vi "Configure Numeric Control.vi"(8 "error in":errorcluster, 10 "control":refnum<vi>, 11 "Value in":refnum<class "Value.lvclass">) -> (0 "error out":errorcluster, 3 "Value out":refnum<class "Value.lvclass">)   [LabVIEW 2020, in "Value.lvlib" / "Value.lvclass"]
doc: "Set the format, precision and limits of the control from the value metadata"
uses:
  Value.lvclass
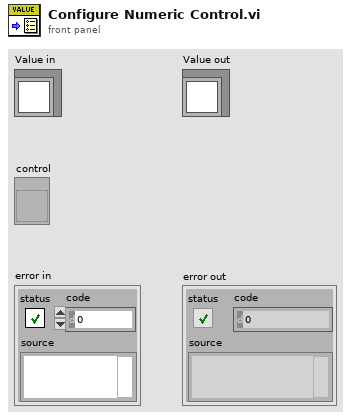
[diagram p1: front panel]
types:
  T1 = typedef "Value.lvlib/Display Metadata.ctl" = cluster{"Limit Low":dbl, "Limit High":dbl, "Description":string, "Units":string, "Precision":i32, "Form":enum32{"Default", "String", "Binary", "Decimal", "Hex", "Exponential", "Engineering"}}
  T2 = enum32{"Default", "String", "Binary", "Decimal", "Hex", "Exponential", "Engineering"}
  T3 = typedef "Value.lvlib/Control Metadata.ctl" = cluster{"Limit Low":dbl, "Limit High":dbl, "Min Step":dbl}
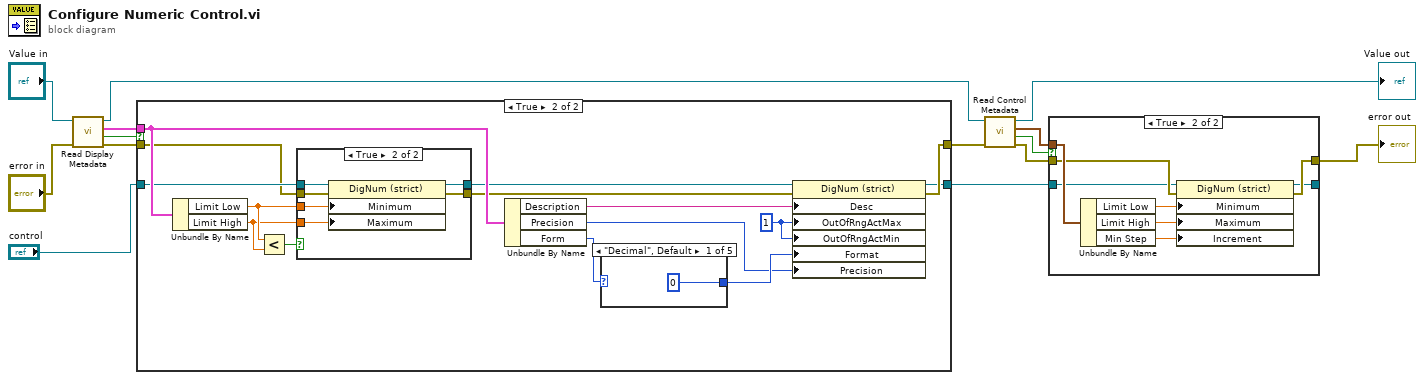
[diagram p0: block diagram]
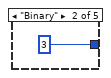
[diagram p5: hidden frame]
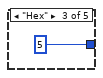
[diagram p6: hidden frame]
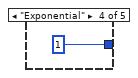
[diagram p7: hidden frame]
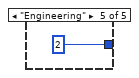
[diagram p8: hidden frame]
diagram:
  n1 = call "Read Display Metadata.vi"("error in"="error in", "Value in"="Value in") -> ("error out"=w10:errorcluster, "has display metadata?"=w7:bool, "display metadata"=w11:T1, "Value out"=w8:refnum<class "Value.lvclass">)  [unwired: 6 in]
  n2 = case shown="True" w7 {
    tunnel: "control" -> [w15 w22]
    tunnel: w11 -> [_ w24]
    tunnel: w10 -> [w16 w20]
    tunnel: [w16 w26] -> w9
    tunnel: [w15 w25] -> w1
    frame False {
    }
    frame True {
      w29 = u8 1 ("Response to Value Outside Limits:Maximum")
      n3 = Unbundle By Name(w24) -> ("Limit Low"=w18:dbl, "Limit High"=w17:dbl)
      n4 = Less?(x=w18, y=w17) -> (x < y?=w23:bool)
      n5 = case shown="True" w23 {
        tunnel: w22 -> [w33 w39]
        tunnel: [w33 w38] -> w21
        tunnel: w20 -> [w32 w37]
        tunnel: [w32 w36] -> w19
        tunnel: w18 -> [_ w35]
        tunnel: w17 -> [_ w34]
        frame False {
        }
        frame True {
          n6 = property on="Property Node" class="DigNum (strict)"(reference=w39, error in=w37, "Minimum"=w35, "Maximum"=w34) -> (reference out=w38:refnum<vi>, error out=w36:errorcluster)
        }
      }
      n7 = Unbundle By Name(w24) -> ("Description"=w30:string, "Precision"=w27:i32, "Form"=w31:T2)
      n8 = case shown="\"Decimal\", Default" w31 {
        tunnel: [u8 0 u8 3 u8 5 u8 1 u8 2] -> w28
        frame "Decimal", Default {
        }
        frame "Binary" {
        }
        frame "Hex" {
        }
        frame "Exponential" {
        }
        frame "Engineering" {
        }
      }
      n9 = property on="Property Node" class="DigNum (strict)"(reference=w21, error in=w19, "Desc"=w30, "OutOfRngActMax"=w29, "OutOfRngActMin"=w29, "Format"=w28, "Precision"=w27) -> (reference out=w25:refnum<vi>, error out=w26:errorcluster)
    }
  }
  n10 = call "Read Control Metadata.vi"("error in"=w9, "Value in"=w8) -> ("error out"=w6:errorcluster, "has control metadata?"=w5:bool, "control metadata"=w4:T3, "Value out"=→"Value out":refnum<class "Value.lvclass">)  [unwired: 6 in]
  n11 = case shown="True" w5 {
    tunnel: w4 -> [_ w52]
    tunnel: w6 -> [w46 w51]
    tunnel: [w46 w50] -> w2
    tunnel: w1 -> [w45 w48]
    tunnel: [w45 w47] -> _
    frame False {
    }
    frame True {
      n12 = Unbundle By Name(w52) -> ("Limit Low"=w54:dbl, "Limit High"=w53:dbl, "Min Step"=w49:dbl)
      n13 = property on="Property Node" class="DigNum (strict)"(reference=w48, error in=w51, "Minimum"=w54, "Maximum"=w53, "Increment"=w49) -> (reference out=w47:refnum<vi>, error out=w50:errorcluster)
    }
  }
  "error out" <- w2
